vi "Find Driver Paths.vi"(7 "Re-scan for classes(F)":bool, 8 "error in (no error)":errorcluster) -> (0 "error out":errorcluster, 2 "Driver Names":string[](array[string]), 3 "Driver Paths":path[](array[path]))   [LabVIEW 2020, in "Instrument Detection.lvlib"]
doc: "Get the paths to all drivers in lvlibps at path."
uses:
  Instrument Detection.lvlib
  PPL/HDH.Actor Framework.Core.Utility.lvlibp
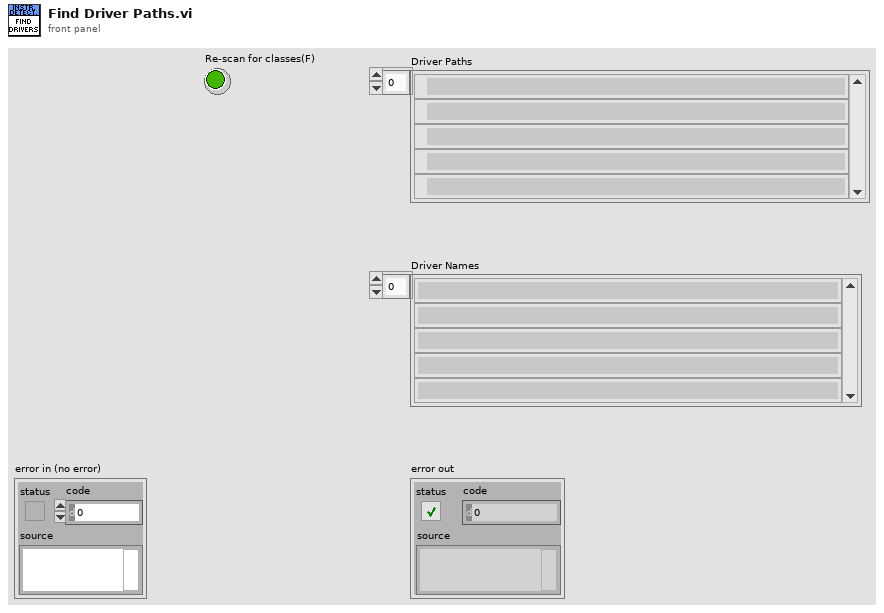
[diagram p1: front panel]
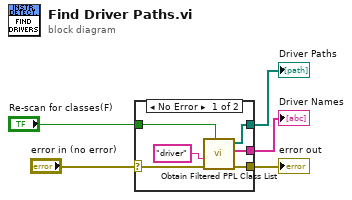
[diagram p0: block diagram]
diagram:
  n1 = case shown="No Error" "error in (no error)" {
    selector: "error in (no error)" -> [w9 w12]
    tunnel: [w7 w12] -> w4
    tunnel: "Re-scan for classes(F)" -> [w11 _]
    tunnel: [w8 _] -> w2
    tunnel: [w6 _] -> w1
    frame No Error {
      n2 = call "Obtain Filtered PPL Class List.vi"("Force reload?(F)"=w11, "error in"=w9, "Post-fix filter(\"\")"="driver" ("Extraction postfix \nWithout .lvclass\ncase insensitive")) -> ("error out"=w7:errorcluster, "PPL Class File Names"=w6:string[], "PPL Class Paths"=w8:path[])  [unwired: 6 in]
    }
    frame Error {
    }
  }
  "error out" <- w4
  "Driver Paths" <- w2
  "Driver Names" <- w1
